vi "LVFunction_Imop_Compute_ModalCoef.vi"(0 "HasoData.lvclass":refnum<class "HasoData.lvclass">, 5 "ComputePhaseSet.lvclass":refnum<class "ComputePhaseSet.lvclass">, 7 "ModalCoef.lvclass":refnum<class "ModalCoef.lvclass">, 11 "error constant":errorcluster) -> (4 "HasoData.lvclass (dup)":refnum<class "HasoData.lvclass">, 6 "ComputePhaseSet.lvclass (dup)":refnum<class "ComputePhaseSet.lvclass">, 8 "ModalCoef.lvclass (dup)":refnum<class "ModalCoef.lvclass">, 15 "error out":errorcluster)   [LabVIEW 2020]
doc: "Compute modal coefficients that represent slopes in a given basis of\npolynomials provided by ComputePhaseSet.\n\n--------------------------------------------------------------------------------\n\nHasoDataIn\n HasoData object.\n\nHasoDataOut\n HasoData object.\n\nComputePhaseSet\n cComputePhaseSet object.\n\nmodalCoef\n cModalCoef object.\n\nErrorIn\n Error\nErrorOut\n Error"
uses:
  HasoData.lvclass
  ComputePhaseSet.lvclass
  ModalCoef.lvclass
  LVClass_ModalCoef Read ModalCoef.vi
  LVClass_ComputePhaseSet Read ComputePhaseSet.vi
  LVClass_HasoData Read HasoData - property.vi
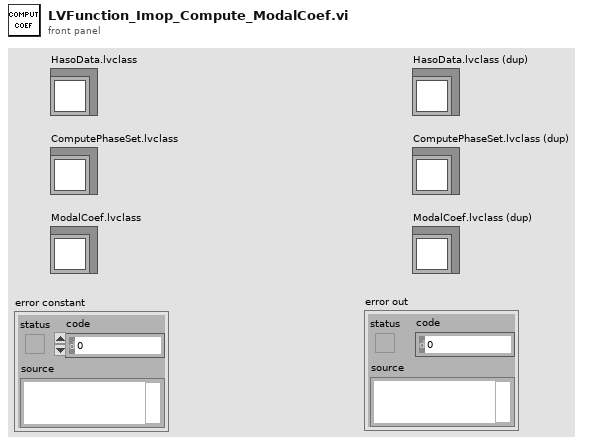
[diagram p1: front panel]
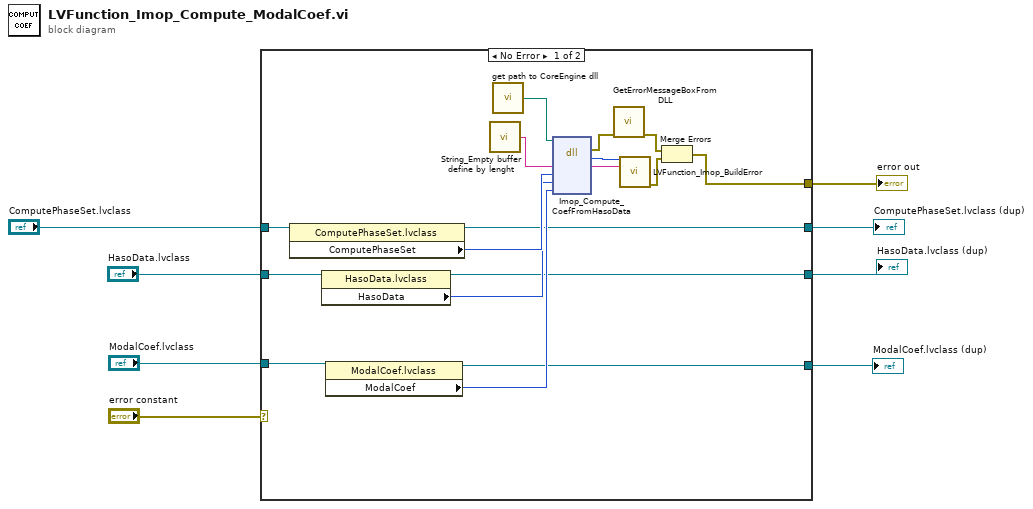
[diagram p0: block diagram]
diagram:
  n1 = case shown="No Error" "error constant" {
    selector: "error constant" -> [_ w29]
    tunnel: "HasoData.lvclass" -> [w20 w27]
    tunnel: "ComputePhaseSet.lvclass" -> [w19 w28]
    tunnel: [w12 w29] -> w7
    tunnel: "ModalCoef.lvclass" -> [w16 w26]
    tunnel: [w11 w26] -> w3
    tunnel: [w10 w27] -> w2
    tunnel: [w9 w28] -> w1
    frame No Error {
      n2 = property class="ComputePhaseSet.lvclass"(reference=w19) -> (reference out=w9:refnum<class "ComputePhaseSet.lvclass">, "ComputePhaseSet"=w18:i32)  [unwired: 1 in, 1 out]
      n3 = property class="HasoData.lvclass"(reference=w20) -> (reference out=w10:refnum<class "HasoData.lvclass">, "HasoData"=w17:i32)  [unwired: 1 in, 1 out]
      n4 = property class="ModalCoef.lvclass"(reference=w16) -> (reference out=w11:refnum<class "ModalCoef.lvclass">, "ModalCoef"=w15:u32)  [unwired: 1 in, 1 out]
      n5 = call "String_Empty buffer define by lenght.vi"() -> ("Empty buffer"=w23:string)  [unwired: 1 in]
      n6 = call "get path to CoreEngine dll.vi"() -> ("path to c_interface_vc100.dll"=w22:path)  [unwired: 12 in, 3 out]
      n7 = dll-call lib="D:/FLE/0.Code/CoreEngine4_Suite/LV2011_interface/DLLs/c_interface_vc100.dll" fn="Imop_Compute_CoefFromHasoData"(path in=w22, "message"=w23, "ComputePhaseSet"=w18, "HasoData"=w17, "ModalCoeffs"=w15) -> (error out=w21:errorcluster, "return type"=w25:i32, "message"=w24:string)  [unwired: 5 in, 1 out]
      n8 = call "GetErrorMessageBoxFromDLL.vi"("error IN"=w21) -> ("error OUT"=w14:errorcluster)  [unwired: 10 in]
      n9 = call "LVFunction_Imop_BuildError.vi"("code"=w25, "String to Prepend to source (\"\")"=w24) -> ("error out"=w13:errorcluster)  [unwired: 13 in]
      n10 = Merge Errors(w14, w13) -> (w12:errorcluster)
    }
    frame Error {
    }
  }
  "error out" <- w7
  "ModalCoef.lvclass (dup)" <- w3
  "HasoData.lvclass (dup)" <- w2
  "ComputePhaseSet.lvclass (dup)" <- w1
